vi "Message Loop Timing.vi"(8 "error in (no error)":errorcluster, 11 "OBS in":refnum<class "OBS.lvclass">) -> (0 "error out":errorcluster, 3 "OBS out":refnum<class "OBS.lvclass">, 4 "Next Timeout":i32)   [LabVIEW 2020, in "obs-websocket.lvlib" / "OBS.lvclass"]
uses:
  OBS.lvclass
  OBS.lvclass/OBS.ctl
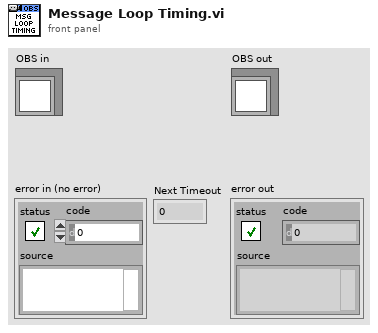
[diagram p1: front panel]
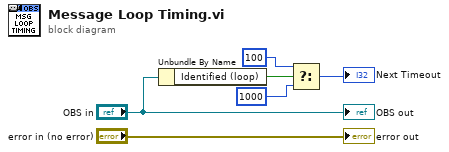
[diagram p0: block diagram]
diagram:
  n1 = Unbundle By Name("OBS in") -> ("Identified (loop)"=w4:bool)
  n2 = Select(t=100, s=w4, f=1000) -> (s? t:f=→"Next Timeout":i32)
  "error out" <- "error in (no error)"
  "OBS out" <- "OBS in"
